vi "Modbus Analyze SRI.vi"(8 "error in":errorcluster, 11 "SRI Butane Values":string[][](array[string])) -> (0 "error out":errorcluster, 3 "Higher than .9% butane":bool)   [LabVIEW 2023, in "Modbus.lvlib"]
uses:
  Modbus.lvlib
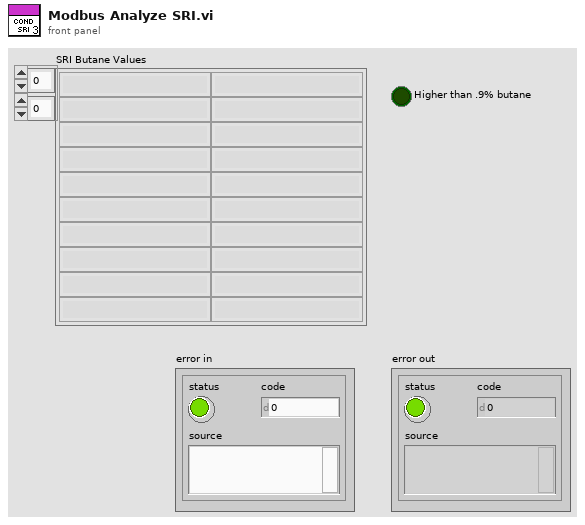
[diagram p1: front panel]
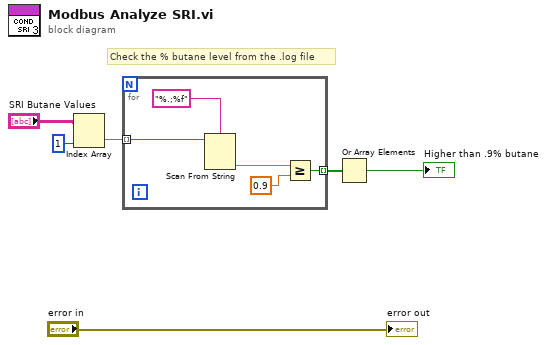
[diagram p0: block diagram]
diagram:
  # "Check the % butane level from the .log file"
  n1 = Index Array(array="SRI Butane Values", index (col)=1 ("disabled index (col)")) -> (element=w2:string[])  [unwired: 1 in]
  n2 = for {
    tunnel: w2 -> [w10] mode=indexing
    tunnel: [w7] -> w6 mode=indexing
    n3 = Scan From String(format string="%.;%f", input string=w10) -> (output 1=w9:dbl)  [unwired: 3 in, 3 out]
    n4 = Greater Or Equal?(x=w9, y=0.9) -> (x >= y?=w7:bool)
  }
  n5 = Or Array Elements(Boolean array=w6) -> (logical OR=→"Higher than .9% butane":bool)
  "error out" <- "error in"
